vi "Example - Caller is not JKISM++.vi"() -> ()   [LabVIEW 2014]
uses:
  user.lib/_NEVSTOP/JKI State Machine ++/Build State String with Arguments++.vi
  user.lib/_NEVSTOP/JKI State Machine ++/Utility/uuid.vi
  user.lib/_NEVSTOP/JKI State Machine ++/Utility/Trim Both Whitespace.vi
  user.lib/_NEVSTOP/JKI State Machine ++/_Support/JKISMQ/_JKISMQFGV.vi
  user.lib/_NEVSTOP/JKI State Machine ++/Utility/Build Error Cluster.vi
  user.lib/_NEVSTOP/JKI State Machine ++/Parse State Queue++.vi
  user.lib/_NEVSTOP/JKI State Machine ++/JKI-State-Machine-Plus.lvlib
panel:
  out "Name":string[](array[string])
  in  "DoSth: DoC(error)":bool
  in  "DoSth: DoB":bool
  in  "DoSth: DoA":bool
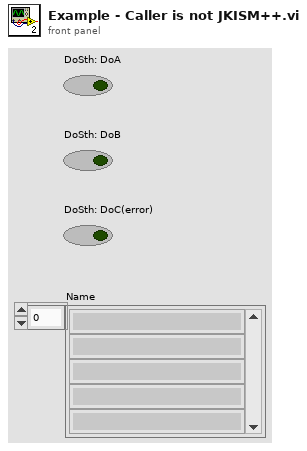
[diagram p1: front panel]
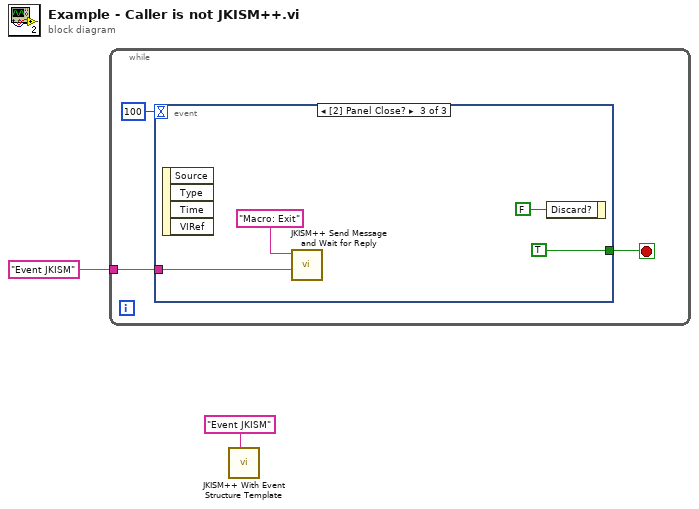
[diagram p0: block diagram]
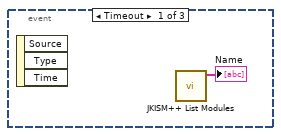
[diagram p2: hidden frame]
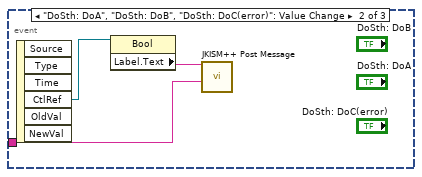
[diagram p3: hidden frame]
diagram:
  n1 = while {
    tunnel: "Event JKISM" ("Name(\"\" to use uuid)") -> [w4]
    stop <- w5 stop-if-true
    n2 = event shown="[2] Panel Close?" {
      selector: _ -> [_ _ _]
      dyn-events: _ -> [_ _ _]
      timeout: 100 -> [_ _ _]
      tunnel: [_ _ TRUE ("Discard?")] -> w5
      tunnel: w4 -> [_ w9 w10]
      event Timeout {
        n3 = event-data() -> ()  [unwired: 1 in, 3 out]
        n4 = call "JKISM++ List Modules.vi"() -> ("Name"=→"Name":string[])  [unwired: 10 in, 1 out]
      }
      event "DoSth: DoA", "DoSth: DoB", "DoSth: DoC(error)": Value Change {
        n5 = event-data() -> ("CtlRef"=w8:refnum<vi>)  [unwired: 1 in, 5 out]
        n6 = property class="Bool"(reference=w8) -> ("Label.Text"=w7:string)  [unwired: 1 in, 2 out]
        n7 = call "JKISM++ Post Message.vi"("Target Module"=w9, "States"=w7) -> ()  [unwired: 9 in, 1 out]
      }
      event Panel Close? {
        n8 = event-data() -> ()  [unwired: 1 in, 4 out]
        n9 = call "JKISM++ Send Message and Wait for Reply.vi"("Target Module"=w10, "States"="Macro: Exit") -> ()  [unwired: 8 in, 2 out]
        n10 = event-data("Discard?"=FALSE) -> ()  [unwired: 1 in, 1 out]
      }
    }
  }
  n11 = call "JKISM++ With Event Structure Template.vi"("Name(\"\" to use uuid)"="Event JKISM" ("Name(\"\" to use uuid)")) -> ()  [unwired: 11 in]
